vi "globalSetUp.vi"(8 "error in (no error)":errorcluster, 11 "MyFirstTest in":refnum<class "MyFirstTest.lvclass">) -> (0 "error out":errorcluster, 3 "MyFirstTest out":refnum<class "MyFirstTest.lvclass">)   [LabVIEW 2013, in "MyFirstTest.lvclass"]
uses:
  MyFirstTest.lvclass
panel:
  out "created new?":bool
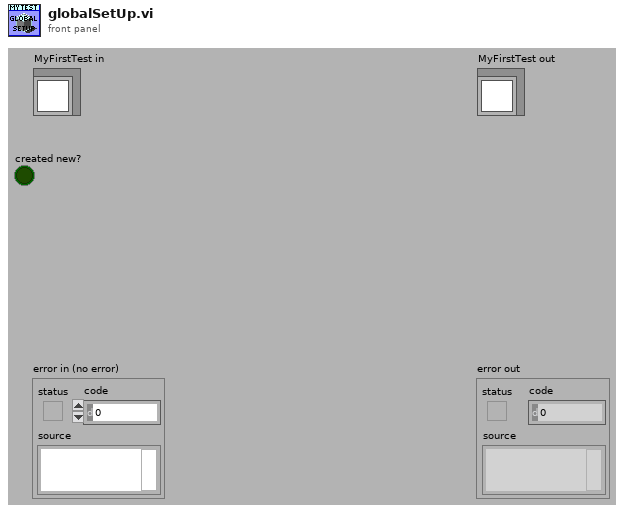
[diagram p1: front panel]
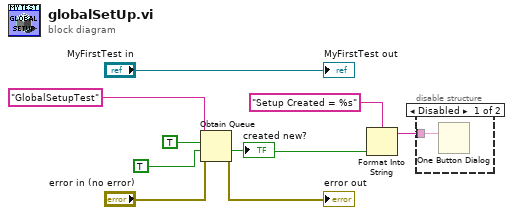
[diagram p0: block diagram]
diagram:
  n1 = Obtain Queue(name (unnamed)="GlobalSetupTest", element data type=TRUE, create if not found? (T)=TRUE, error in (no error)="error in (no error)") -> (created new?=w3:bool, error out=→"error out":errorcluster)  [unwired: 1 in, 1 out]
  "created new?" <- w3
  n2 = Format Into String(format string="Setup Created = %s", w3) -> (resulting string=w2:string)  [unwired: 2 in, 1 out]
  n3 = disable-structure shown="Disabled" {
    disable-tunnel: w2 -> [w10 _]
    frame Disabled {
      n4 = One Button Dialog(message=w10) -> ()  [unwired: 1 in, 1 out]
    }
    frame Enabled {
    }
  }
  "MyFirstTest out" <- "MyFirstTest in"
